vi "Simulated Robot Example 1.vi"() -> ()   [LabVIEW 2019]
doc: "This VI demonstrates how to control a simulated Robotics Starter Kit 2.0 robot. With a few modifications, you can deploy this VI to the Single-Board RIO 9632 on a real robot, and it runs on the real-time controller. For more information about how to modify this VI so you can deploy it to real hardware, refer to the <B>Robotics Module>>Simulating Mobile Robots</B> book on the <B>Contents</B> tab of the LabVIEW Help."
uses:
  <vilib>/robotics/Simulator/Engine/ctl/Step Mode.ctl
  <vilib>/robotics/Simulator/Engine/ctl/Simulation Mode.ctl
  <vilib>/Platform/TimedLoop/XDataNode/timing_clust.ctl
  <vilib>/Platform/TimedLoop/XDataNode/nitl_modes.ctl
  <vilib>/Platform/TimedLoop/XDataNode/wakeup.ctl
  Stage_var.vi
  Init_var.vi
  Sequence_var.vi
  Scanned.vi
  Arm_stage_var.vi
  Mashina_podyehala.vi
  Camera_angle.vi
  Color_num_var.vi
  Ball_num_var.vi
  Completed_var.vi
  Global_count_var.vi
  <vilib>/robotics/Simulator/Interface/Simulator References/Get 3D Visual Scene Reference.vi
  <vilib>/Platform/TimedLoop/XDataNode/XDataNode.xnode
  <vilib>/robotics/Simulator/NI_Robotics_Simulator.lvlib
  <vilib>/Platform/TimedLoop/XDataNode/XDNodeRunTimeDep.lvlib
  Simulation SubVIs/Simulation SubVIs.lvlib
panel:
  in  "Panelka port":u16
  in  "Env port":u16
  out "CameraScene":refnum<vi>(3d-picture)
  out "error out":errorcluster
  in  "stop":bool
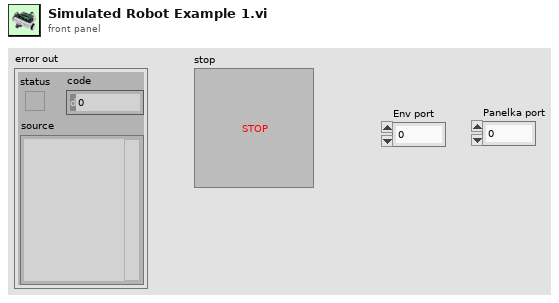
[diagram p1: front panel]
types:
  T1 = typedef "XDNodeRunTimeDep.lvlib/timing_clust.ctl" = cluster{"Expected End [f-1]":u64, "Actual End [f-1]":u64, "Finished Late? [f-1]":bool, "Expected End [i-1]":u64, "Actual End [i-1]":u64, "Finished Late? [i-1]":bool, "Expected Start [i]":u64, "Actual Start [i]":u64, "Expected Start [f]":u64, "Actual Start [f]":u64, "Source Name":string, "Structure Name":string, "Period":i64, "Deadline":i64, "Offset":i64, "Start":i64, "Priority":i32, "Timeout":i32, "Mode":T2, "Wakeup Reason":T3, "Error":errorcluster, "Source Type":string, "Secondary Source Type":string, "Global End Time":u64, "Global Start Time":u64, "Frame Duration":u64, "Iteration Duration":u64, "Assigned CPU":i32, "I/O Scan Engine Mode":u32}
  T2 = typedef "XDNodeRunTimeDep.lvlib/nitl_modes.ctl" = enum32{"No Change", "Process missed periods, maintain original phase", "Discard missed periods, maintain original phase", "Process missed periods, ignore original phase", "Discard missed periods, ignore original phase"}
  T3 = typedef "XDNodeRunTimeDep.lvlib/wakeup.ctl" = enum32{"Normal", "Aborted", "Asynchronous wakeup", "Timing source error", "Timed loop error", "Timeout"}
  T4 = typedef "Image Type" = u32
  T5 = typedef "NI_Robotics_Simulator.lvlib/Simulation Mode.ctl" = u16
  T6 = typedef "NI_Robotics_Simulator.lvlib/Step Mode.ctl" = u16
  T7 = typedef "IMAQ Image.ctl" = refnum<image>
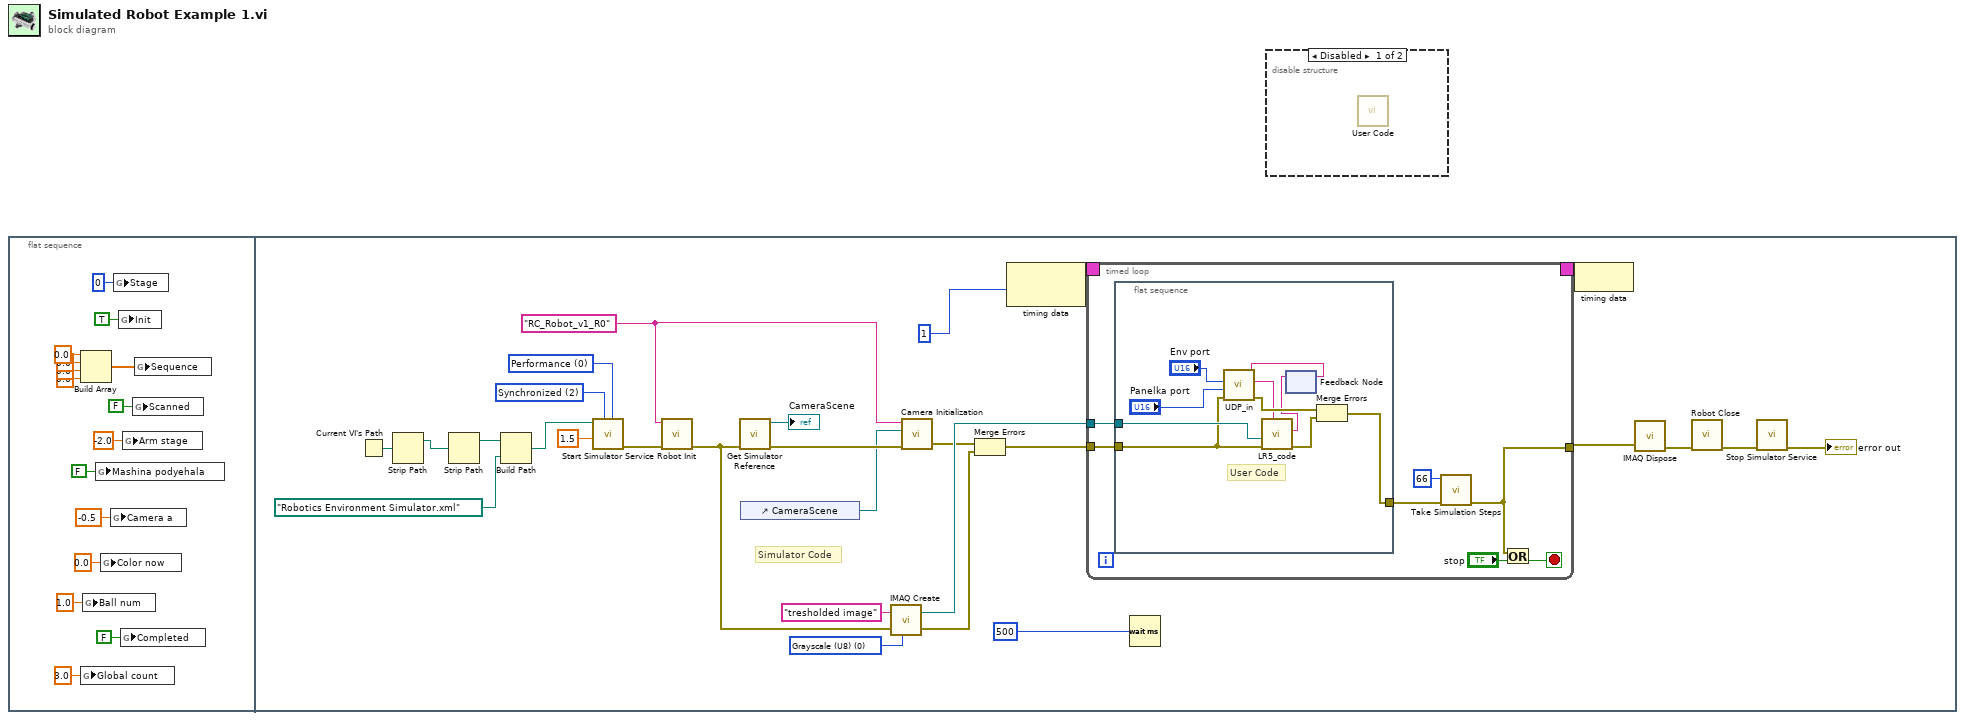
[diagram p0: block diagram]
diagram:
  n1 = flat-sequence {
    frame #0 {
      n2 = Build Array(0.0 ("element"), 0.0 ("element"), 0.0 ("element"), 0.0 ("element")) -> (w13:dbl[])
      n3 = global write "Global_count_var.vi" "Global count"(3.0 ("Global count")) -> ()
      n4 = global write "Ball_num_var.vi" "Ball num"(1.0 ("Ball num")) -> ()
      n5 = global write "Mashina_podyehala.vi" "Mashina podyehala"(FALSE ("Mashina podyehala")) -> ()
      n6 = global write "Color_num_var.vi" "Color now"(0.0 ("Color now")) -> ()
      n7 = global write "Camera_angle.vi" "Camera a"(-0.5 ("Camera a")) -> ()
      n8 = global write "Stage_var.vi" "Stage"(u32 0 ("Stage")) -> ()
      n9 = global write "Init_var.vi" "Init"(TRUE ("Init")) -> ()
      n10 = global write "Completed_var.vi" "Completed"(FALSE ("Completed")) -> ()
      n11 = global write "Arm_stage_var.vi" "Arm stage"(-2.0 ("Arm stage")) -> ()
      n12 = global write "Scanned.vi" "Scanned"(FALSE ("Scanned")) -> ()
      n13 = global write "Sequence_var.vi" "Sequence"(w13) -> ()
    }
    frame #1 {
      w25 = T4 0 items=["Grayscale (U8)", "Grayscale (I16)", "Grayscale (SGL)", "Complex (CSG)", "RGB (U32)", "HSL (U32)", "RGB (U64)", "Grayscale (U16)"] ("Image Type")
      w26 = "RC_Robot_v1_R0" ("robot ID")
      w33 = T5 2 items=["Software Real-Time", "Free Running", "Synchronized"] ("timing mode")
      w35 = T6 0 items=["Performance", "Accuracy"] ("step mode")
      # "Simulator Code"
      n14 = Current VI's Path() -> (path=w40:path)
      n15 = Strip Path(path=w40) -> (stripped path=w39:path)  [unwired: 1 out]
      n16 = Strip Path(path=w39) -> (stripped path=w38:path)  [unwired: 1 out]
      n17 = Build Path(base path=w38, name or relative path=path "Robotics Environment Simulator.xml" ("Simulation Manifest File")) -> (appended path=w36:path)
      n18 = call <vilib>:"Start Simulator Service.vi"("step mode"=w35, "timing mode"=w33, "step size (ms)"=1.5, "manifest file"=w36) -> ("error out"=w29:errorcluster)  [unwired: 7 in]
      n19 = call "Robot Init.vi"("error in (no error)"=w29, "robot ID"=w26) -> ("error out"=w17:errorcluster)  [unwired: 9 in]
      n20 = call-poly <vilib>:"Get Simulator Reference.vi"("error in"=w17) -> ("error out"=w28:errorcluster, "scene ref"=→"CameraScene":refnum<vi>)  [unwired: 9 in]
      n21 = control-ref of="CameraScene"() -> (w27:refnum<vi>)
      n22 = call "IMAQ Create"("Image Name"="tresholded image", "Image Type"=w25, "error in (no error)"=w17) -> ("New Image"=w23:T7, "error out"=w20:errorcluster)  [unwired: 2 in]
      n23 = call "Camera Initialization.vi"("error in (no error)"=w28, "SceneGraphDisplay in"=w27, "robot ID"=w26) -> ("error out"=w21:errorcluster)  [unwired: 8 in]
      n24 = Merge Errors(w21, w20) -> (w22:errorcluster)
      n25 = node-c288(i64 1 ("Period")) -> (w43:T1)
      n26 = timed-loop {
        timing: w43 -> [_]
        timing-out: [_] -> w42
        tunnel: [w47] -> w18
        tunnel: w22 -> [w46]
        tunnel: w23 -> [w45]
        stop <- w49 stop-if-true
        n27 = flat-sequence {
          tunnel: w46 -> [w58]
          tunnel: w45 -> [w60]
          tunnel: [w57] -> w44
          frame #0 {
            # "User Code"
            n28 = feedback #1() -> (w51:string)  [unwired: 1 in]
            n29 = call "UDP_in.vi"("data in"=w51, "error in (no error)"=w58, "Panelka port"="Panelka port", "Env port"="Env port") -> ("error out"=w56:errorcluster, "data out"=w54:string)  [unwired: 6 in]
            n30 = call "LR5_code.vi"("data in"=w54, "error in (no error)"=w58, "Image Dst"=w60) -> ("error out"=w55:errorcluster, "data out"=w52:string)  [unwired: 7 in]
            n31 = feedback-in #1(w52) -> ()
            n32 = Merge Errors(w56, w55) -> (w57:errorcluster)
          }
        }
        n33 = call <vilib>:"Take Simulation Steps.vi"("error in (no error)"=w44, "number of steps"=u64 66) -> ("error out"=w47:errorcluster)  [unwired: 9 in]
        n34 = Or(x=w47, y="stop") -> (x .or. y?=w49:bool)
      }
      n35 = Wait (ms)(milliseconds to wait=u32 500) -> ()  [unwired: 1 out]
      n36 = node-c288(w42) -> ()
      n37 = call "IMAQ Dispose"("error in (no error)"=w18) -> ("error out"=w19:errorcluster)  [unwired: 5 in]
      n38 = call "Robot Close.vi"("error in (no error)"=w19) -> ("error out"=w31:errorcluster)  [unwired: 10 in]
      n39 = call <vilib>:"Stop Simulator Service.vi"("error in (no error)"=w31) -> ("error out"=→"error out":errorcluster)  [unwired: 10 in]
    }
  }
  n40 = disable-structure shown="Disabled" {
    frame Disabled {
      n41 = call "User Code.vi"() -> ()  [unwired: 11 in, 1 out]
    }
    frame Enabled {
    }
  }
